vi "Sensirion SHT25 - VISA set IO pins.vi"(8 "Error In":errorcluster, 10 "I/O pins":string="\u0000", 11 "VISA in":refnum<visa-resource-name>) -> (0 "Error Out":errorcluster, 1 "read buffer":string, 3 "VISA out":refnum<visa-resource-name>)   [LabVIEW 2012]
uses:
  Sensirion SHT25 - USB-I2C primary command.ctl
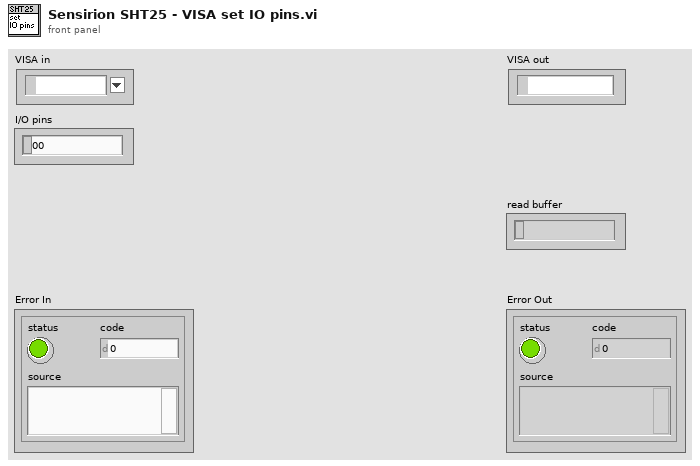
[diagram p1: front panel]
types:
  T1 = typedef "Sensirion SHT25 - USB-I2C primary command.ctl" = u8
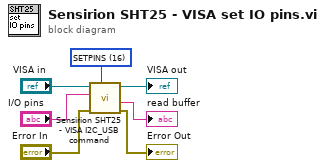
[diagram p0: block diagram]
diagram:
  w6 = T1 16 items=["REVISION"=1, "NEW ADDRESS"=2, "SCAN1"=4, "SCAN2"=5, "SCAN3"=6, "SCAN4"=7, "SCAN6"=8, "SCAN8"=9, "SCAN12"=10, "SCAN16"=11, "SETPINS"=16, "GETPINS"=17, "GETAD"=18] ("command")
  n1 = call "Sensirion SHT25 - VISA I2C_USB command.vi"("command"=w6, "Error In"="Error In", "data 1"="I/O pins", "VISA in"="VISA in") -> ("Error Out"=→"Error Out":errorcluster, "read buffer"=→"read buffer":string, "VISA out"=→"VISA out":refnum<visa-resource-name>)  [unwired: 5 in]
